vi "Main.vi"() -> ()   [LabVIEW 2017]
doc: "The myRIO Project template acquires acceleration data from the onboard accelerometer and displays the changes of acceleration values in a waveform chart."
uses:
  <vilib>/myRIO/Instrument Drivers/Onboard IO/PWM/typedefs/PWM Reference.ctl
  <vilib>/myRIO/Common/Instrument Driver Framework/Utilities/typedefs/myRIO Generic Hardware Reference.ctl
  <vilib>/myRIO/Common/Instrument Driver Framework/Utilities/typedefs/Hardware Version Enum.ctl
  <vilib>/myRIO/Common/Instrument Driver Framework/Utilities/typedefs/myRIO v1.0 Reference.ctl
  <vilib>/myRIO/Common/Instrument Driver Framework/Utilities/typedefs/Generic FPGA Reference.ctl
  <vilib>/myRIO/Common/Instrument Driver Framework/myRIO v1.0/PWM/typedefs/PWM Channels Enum.ctl
  <vilib>/myRIO/Instrument Drivers/Onboard IO/PWM/typedefs/PWM Configuration.ctl
  <vilib>/myRIO/Instrument Drivers/Onboard IO/AI/typedefs/AI Reference.ctl
  <vilib>/myRIO/Common/Instrument Driver Framework/myRIO v1.0/AI/typedefs/AI Channels List.ctl
  <vilib>/myRIO/Common/Instrument Driver Framework/myRIO v1.0/AI/typedefs/AI Channels Enum.ctl
  <vilib>/myRIO/Common/Instrument Driver Framework/Utilities/typedefs/Analog Scaling Constants List.ctl
  <vilib>/myRIO/Common/Instrument Driver Framework/Utilities/typedefs/Analog Scaling Constants.ctl
  <vilib>/userdefined/High Color/nirio_resource_hc.ctl
  <vilib>/myRIO/Common/Instrument Driver Framework/Utilities/vis/Is FPGA Ref Available.vi
  <vilib>/myRIO/Common/Instrument Driver Framework/myRIO v1.0/AI/vis/myRIO v1.1 Open AI.vi
  <vilib>/myRIO/Instrument Drivers/Onboard IO/AI/vis/Read.vi
  <vilib>/myRIO/Common/Instrument Driver Framework/myRIO v1.0/PWM/vis/myRIO v1.1 Open PWM.vi
  <vilib>/myRIO/Common/Instrument Driver Framework/Utilities/vis/Validate Channels.vi
  <vilib>/myRIO/Common/Instrument Driver Framework/myRIO v1.0/AI/vis/myRIO v1.0 Reserve AI.vi
  <vilib>/myRIO/Common/Instrument Driver Framework/myRIO v1.0/UART/vis/myRIO v1.0 Close UART.vi
  <vilib>/myRIO/Common/Instrument Driver Framework/myRIO v1.0/PWM/vis/myRIO v1.0 Reserve PWM.vi
  <vilib>/myRIO/Common/Instrument Driver Framework/myRIO v1.0/AI/vis/myRIO v1.0 Build MUX Configuration AI.vi
  <vilib>/myRIO/Common/Instrument Driver Framework/myRIO v1.0/Resource Manager/vis/myRIO v1.0 Reserve Channel List.vi
  <vilib>/myRIO/Common/Instrument Driver Framework/myRIO v1.0/PWM/vis/myRIO v1.0 Build MUX Configuration PWM.vi
  <vilib>/myRIO/Common/Instrument Driver Framework/myRIO v1.0/Resource Manager/vis/myRIO v1.0 Reserve Channel.vi
  <vilib>/myRIO/Common/Instrument Driver Framework/myRIO v1.0/Resource Manager/vis/myRIO v1.0 Unreserve Channel.vi
  <vilib>/myRIO/Common/Instrument Driver Framework/myRIO v1.0/Resource Manager/vis/myRIO v1.0 Create Configuration List.vi
  <vilib>/myRIO/Common/Instrument Driver Framework/myRIO v1.0/Resource Manager/vis/myRIO v1.0 Build Mutex Name.vi
  <vilib>/Utility/VariantDataType/GetNumericInfo.vi
  <vilib>/Utility/error.llb/Error Cluster From Error Code.vi
  <vilib>/myRIO/Common/Instrument Driver Framework/myRIO v1.0/myRIO v1.1 Open.vi
  <vilib>/myRIO/Common/Instrument Driver Framework/Utilities/vis/IO Manager.vi
  <vilib>/myRIO/Common/Instrument Driver Framework/Utilities/vis/Configuration Manager.vi
  <vilib>/myRIO/Common/Instrument Driver Framework/myRIO v1.0/Resource Manager/vis/myRIO v1.0 Configure IO.vi
  <vilib>/myRIO/Common/Instrument Driver Framework/myRIO v1.0/myRIO v1.0 Close.vi
  <vilib>/myRIO/Common/Instrument Driver Framework/myRIO v1.0/AI/vis/myRIO v1.0 Get Scaling Constants AI.vi
  <vilib>/myRIO/Common/Instrument Driver Framework/myRIO v1.0/AI/vis/myRIO v1.0 Read AI.vi
  <vilib>/myRIO/Common/Instrument Driver Framework/myRIO v1.0/PWM/vis/myRIO v1.0 Write PWM.vi
  <vilib>/myRIO/Common/Instrument Driver Framework/Utilities/vis/FPGA Ref Manager.vi
  <vilib>/myRIO/Common/Instrument Driver Framework/myRIO v1.0/myRIO v1.0 Reset FPGA.vi
  <vilib>/myRIO/Common/Instrument Driver Framework/myRIO v1.0/IRQ/vis/myRIO v1.0 IRQ Info FGV.vi
  <vilib>/myRIO/Common/Instrument Driver Framework/myRIO v1.0/IRQ/vis/myRIO v1.0 Timer IRQ Info FGV.vi
  <vilib>/myRIO/Common/Instrument Driver Framework/myRIO v1.0/IRQ/vis/myRIO v1.0 ISR Agent.vi
  <vilib>/myRIO/Express VI/Onboard IO/AI/AI Express VI.xnode
  <vilib>/myRIO/Instrument Drivers/Onboard IO/AI/vis/myRIO AI Open.xnode
  <vilib>/myRIO/Instrument Drivers/Utilities/Utilities.lvlib
  <vilib>/myRIO/Instrument Drivers/Onboard IO/AI/AI.lvlib
  <vilib>/myRIO/Instrument Drivers/Onboard IO/PWM/PWM.lvlib
panel:
  in  "PWM Ref Out":T1
  out "Pre-Set Frequency":dbl
  out "error out 2":errorcluster
  out "offset [%FS]":dbl
  in  "null offset 2":bool
  out "duty cycle [%] 2":dbl
  out "pulse width [ms] 2":dbl=1.5
  in  "position [%FS] 2":dbl(slide) scale=-200.0..200.0
  in  "PWM channel":tag="B/PWM0"
  out "Current":dbl
  out "error out":errorcluster
  in  "Stop":bool
  # "Overview: The myRIO Project template acquires acceleration data from the onboard accelerometer and displays the changes of acceleration values in a waveform chart.\nInstructions:\n1. Check the myRIO target IP address in the project and make sure the target IP address is correct. \n2. Run this VI."
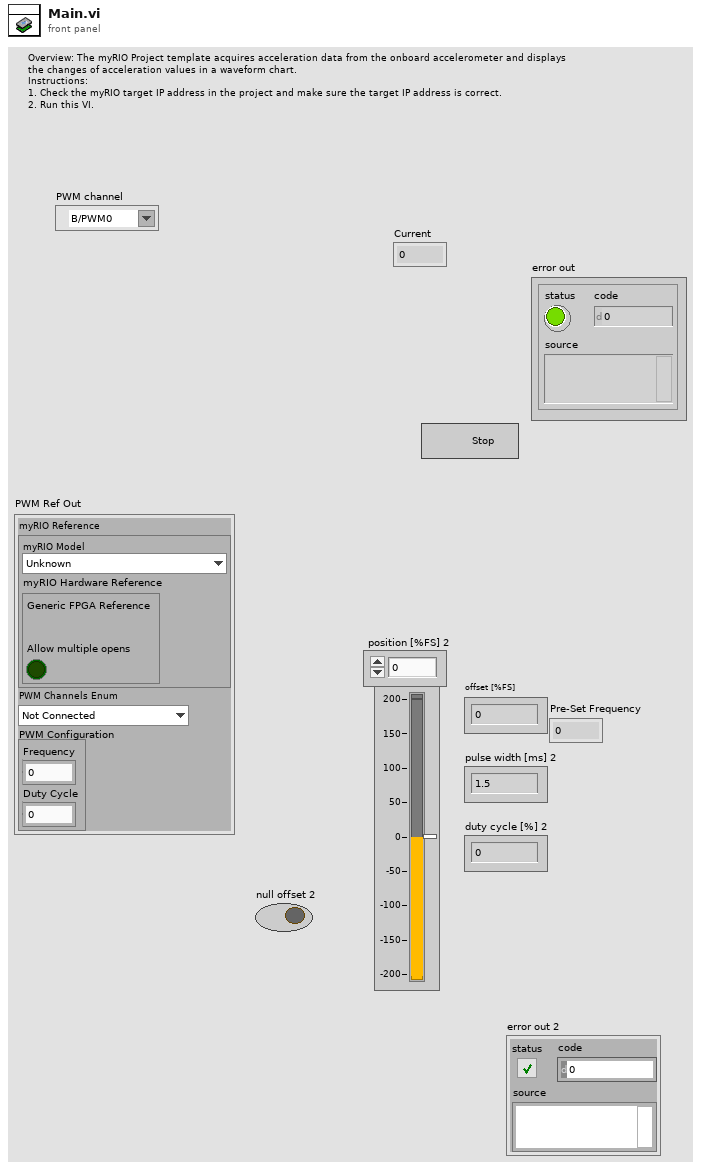
[diagram p1: front panel]
types:
  T1 = typedef "PWM.lvlib/PWM Reference.ctl" = cluster{"myRIO Reference":T2, "PWM Channels Enum":T6, "PWM Configuration":T7}
  T2 = typedef "myRIO Generic Hardware Reference.ctl" = cluster{"myRIO Model":T3, "myRIO Hardware Reference":T4}
  T3 = typedef "Hardware Version Enum.ctl" = enum16{"Unknown", "myRIO-1900", "myRIO-1950", "roboRIO", "NI ELVIS RIO CM"}
  T4 = typedef "myRIO v1.0 Reference.ctl" = cluster{"Generic FPGA Reference":T5, "Allow multiple opens":bool}
  T5 = typedef "Generic FPGA Reference.ctl" = refnum<k20>
  T6 = typedef "PWM Channels Enum.ctl" = enum16{"Not Connected", "C/PWM0", "C/PWM1", "A/PWM0", "A/PWM1", "A/PWM2", "B/PWM0", "B/PWM1", "B/PWM2", "PWM/PWM0", "PWM/PWM1", "PWM/PWM2", "PWM/PWM3", "PWM/PWM4", "PWM/PWM5", "PWM/PWM6", "PWM/PWM7", "PWM/PWM8", "PWM/PWM9"}
  T7 = typedef "PWM.lvlib/PWM Configuration.ctl" = cluster{"Frequency":dbl, "Duty Cycle":dbl}
  T8 = enum16{"open", "replace", "create", "open or create", "replace or create", "replace or create with confirmation"}
  T9 = typedef "AI.lvlib/AI Reference.ctl" = cluster{"myRIO Reference":T2, "AI Channels List":T10, "AI Scaling Constants List":T12}
  T10 = typedef "AI Channels List.ctl" = T11[]
  T11 = typedef "AI Channels Enum.ctl" = enum16{"Not Connected", "AudioIn/Left", "AudioIn/Right", "C/AI0", "C/AI1", "A/AI0", "A/AI1", "A/AI2", "A/AI3", "B/AI0", "B/AI1", "B/AI2", "B/AI3", "AI/AI0", "AI/AI1", "AI/AI2", "AI/AI3"}
  T12 = typedef "Analog Scaling Constants List.ctl" = T13[]
  T13 = typedef "Analog Scaling Constants.ctl" = cluster{"LSB Weight (Volts)":dbl, "Offset (Volts)":dbl, "Signed?":bool}
  T14 = typedef "nirio_resource_hc.ctl" = tag
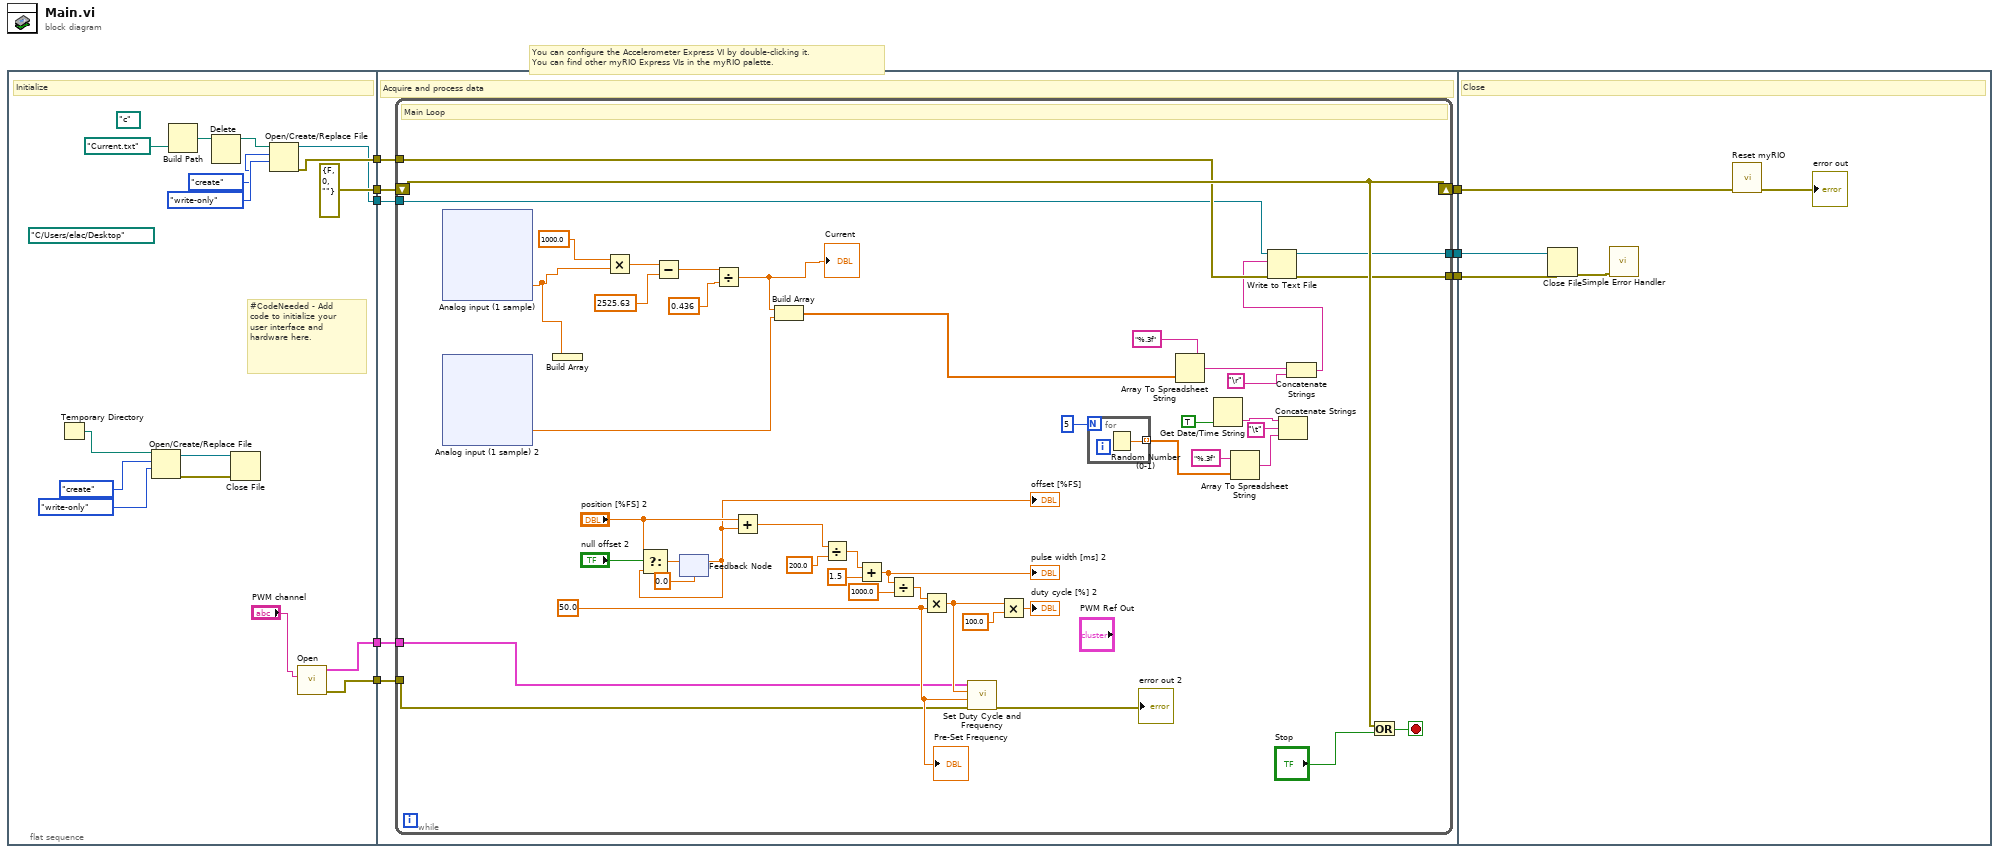
[diagram p0: block diagram]
diagram:
  # "You can configure the Accelerometer Express VI by double-clicking it.\nYou can find other myRIO Express VIs in the myRIO palette."
  n1 = flat-sequence {
    tunnel: [errorcluster {"status"=FALSE, "code"=0, "source"=""} ("error in (no error)")] -> w8
    tunnel: [w23] -> w6
    tunnel: [w21] -> w5
    tunnel: [w15] -> w2
    tunnel: [w14] -> w1
    tunnel: w8 -> [w32]
    tunnel: [w31] -> w7
    tunnel: w6 -> [w30]
    tunnel: w5 -> [w29]
    tunnel: [w28] -> w4
    tunnel: [w27] -> w3
    tunnel: w2 -> [w26]
    tunnel: w1 -> [w25]
    tunnel: w7 -> [w158]
    tunnel: w4 -> [w156]
    tunnel: w3 -> [w155]
    frame #0 {
      (unwired) path "c:/" ("base path")
      (unwired) path "C:/Users/elac/Desktop" ("base path")
      # "#CodeNeeded - Add code to initialize your user interface and hardware here."
      # "Initialize"
      n2 = Temporary Directory() -> (w9:path)
      n3 = Open/Create/Replace File(file path (use dialog)=w9, operation (0:open)=T8."create", access (0:read/write)=enum16{"read/write", "read-only", "write-only"}."write-only") -> (refnum out=w12:refnum<file>, error out=w11:errorcluster)  [unwired: 3 in, 1 out]
      n4 = Build Path(name or relative path=path "Current.txt" ("default name")) -> (appended path=w19:path)  [unwired: 1 in]
      n5 = Delete(path (use dialog)=w19) -> (deleted path=w20:path)  [unwired: 4 in, 2 out]
      n6 = Close File(refnum=w12, error in=w11) -> ()  [unwired: 2 out]
      n7 = Open/Create/Replace File(file path (use dialog)=w20, operation (0:open)=T8."create", access (0:read/write)=enum16{"read/write", "read-only", "write-only"}."write-only") -> (refnum out=w14:refnum<file>, error out=w15:errorcluster)  [unwired: 1 in, 3 out]
      n8 = call <vilib>:"Open.vi"("Channel Name"="PWM channel") -> ("error out"=w23:errorcluster, "PWM Ref Out"=w21:T1)  [unwired: 9 in]
    }
    frame #1 {
      # "Acquire and process data"
      n9 = while {
        shift-right: [w52] -> w31
        shift-left: w32 -> [w52]
        tunnel: w30 -> [w54]
        tunnel: w29 -> [w53]
        tunnel: [w49] -> w28
        tunnel: [w48] -> w27
        tunnel: w26 -> [w47]
        tunnel: w25 -> [w46]
        stop <- w77 stop-if-true
        w55 = 50.0 ("freq [Hz]")
        # "Main Loop"
        n10 = xnode "Analog input (1 sample)"() -> ("A/AI0 (Pin 3)"=w34:dbl)  [unwired: 1 in, 1 out]
        n11 = xnode "Analog input (1 sample) 2"() -> ("A/AI1 (Pin 5)"=w33:dbl)  [unwired: 1 in, 1 out]
        n12 = Build Array(w34) -> ()  [unwired: 1 out]
        n13 = Multiply(x=1000.0, y=w34) -> (x*y=w75:dbl)
        n14 = Subtract(x=w75, y=2525.63) -> (x-y=w73:dbl)
        n15 = feedback #1(0.0 ("position [%FS]")) -> (w65:dbl)
        "offset [%FS]" <- w65
        n16 = Select(t="position [%FS] 2", s="null offset 2", f=w65) -> (s? t:f=w63:dbl)
        n17 = feedback-in #1(w63) -> ()
        n18 = Divide(x=w73, y=0.436) -> (x/y=w50:dbl)
        "Current" <- w50
        n19 = Add(x="position [%FS] 2", y=w65) -> (x+y=w64:dbl)
        n20 = Build Array(w50, w33) -> (w35:dbl[])
        n21 = Divide(x=w64, y=200.0) -> (x/y=w57:dbl)
        n22 = Add(x=w57, y=1.5) -> (x+y=w59:dbl)
        "pulse width [ms] 2" <- w59
        n23 = Divide(x=w59, y=1000.0) -> (x/y=w66:dbl)
        n24 = Multiply(x=w66, y=w55) -> (x*y=w69:dbl)
        n25 = call <vilib>:"Set Duty Cycle and Frequency.vi"("error in (no error)"=w54, "Frequency [Hz]"=w55, "Duty Cycle"=w69, "PWM Ref In"=w53) -> ("error out"=→"error out 2":errorcluster)  [unwired: 5 in, 1 out]
        n26 = Multiply(x=w69, y=100.0) -> (x*y=→"duty cycle [%] 2":dbl)
        n27 = for {
          N: 5 ("number of points/acquisition") -> [_]
          tunnel: [w116] -> w40 mode=indexing
          n28 = Random Number (0-1)() -> (number: 0 to 1=w116:dbl)
        }
        n29 = Array To Spreadsheet String(array=w35, 3:"%.3f") -> (spreadsheet string=w37:string)  [unwired: 1 out]
        n30 = Get Date/Time String(want seconds? (F)=TRUE) -> (time string=w39:string)  [unwired: 2 in, 1 out]
        n31 = Array To Spreadsheet String(array=w40, 3:"%.3f") -> (spreadsheet string=w44:string)  [unwired: 1 out]
        n32 = Concatenate Strings(w39, "\t" ("Tab"), w44) -> ()  [unwired: 1 out]
        n33 = Concatenate Strings(w37, "\r") -> (w38:string)
        n34 = Write to Text File(file (use dialog)=w46, text=w38, error in=w47) -> (refnum out=w49:refnum<file>, error out=w48:errorcluster)  [unwired: 1 in, 1 out]
        n35 = Or(x=w52, y="Stop") -> (x .or. y?=w77:bool)
        "Pre-Set Frequency" <- w55
      }
    }
    frame #2 {
      # "Close"
      n36 = Close File(refnum=w156, error in=w155) -> (error out=w154:errorcluster)  [unwired: 1 out]
      n37 = call <vilib>:"Simple Error Handler.vi"("error in (no error)"=w154) -> ()  [unwired: 1 in, 8 out]
      n38 = call <vilib>:"Reset myRIO.vi"("error in (no error)"=w158) -> ("error out"=→"error out":errorcluster)  [unwired: 10 in]
    }
  }
